vi "Message Update.vi"(8 "error in (no error)":errorcluster, 9 "Replace request":T1, 10 "Message type":string="Message") -> (0 "error out":errorcluster, 2 "Message Out":string)   [LabVIEW 2019]
uses:
  controls/Replace Request.ctl
  controls/Message_type.ctl
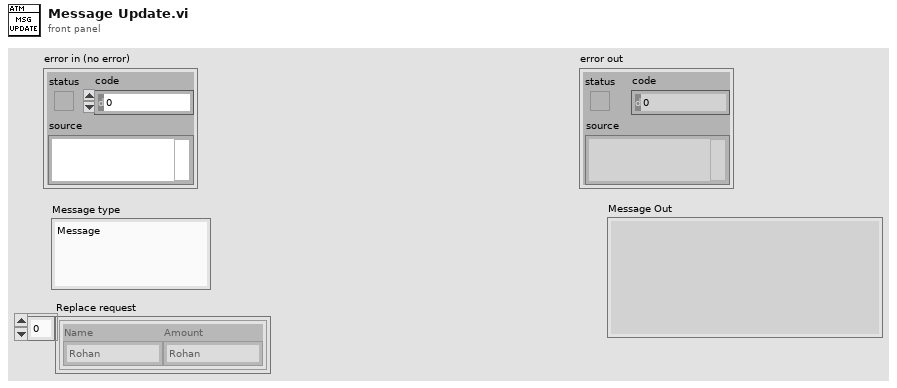
[diagram p1: front panel]
types:
  T1 = typedef "Replace Request.ctl" = cluster{"Name":string, "Amount":string}[]
  T2 = typedef "Message_type.ctl" = string[][]
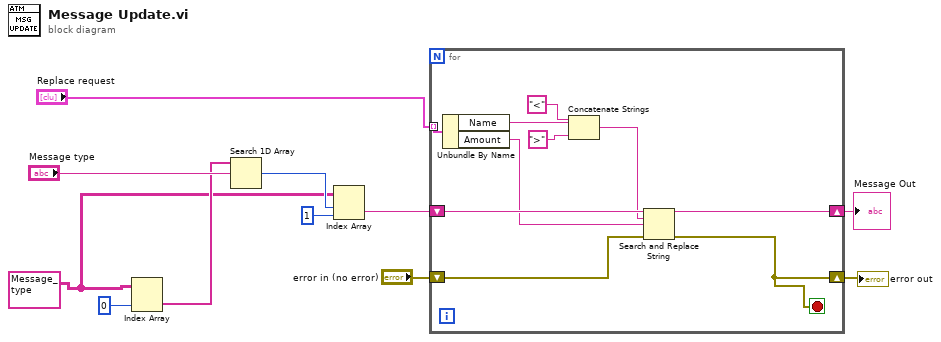
[diagram p0: block diagram]
diagram:
  w1 = T2 [["Welcome", "Welcome to Acme Bank.\nPlease insert your card\nand enter your account\nnumber in the User Input.\n\nPress Enter (E) when done."], ["Main Menu", "Welcome to Acme Bank\n<Name>\n\nPlease select transaction by using the buttons."], ["Account Verification Failed", "Account Information Incorrect.\nPlease Re-Enter Account Number.\nPress Enter (E) when done."], ["Session Terminate", "Your session has been terminated due to inactivity or menu selection.\nPlease take your card.\n\nGoodbye!"], ["Deposit", "Please enter amount to deposit and press Enter (E) when done."], ["Deposit Complete", "<Amount> Deposited"], ["Withdrawal", "Please enter amount to withdraw and press Enter (E) when done."], ["Withdrawal Complete", "<Amount> Withdrawn"], ["Withdrawal Failed", "Insufficient funds in account.\nPlease check your balance and try again."], ["Balance Inquiry", "Your Balance Is:\n<Amount>"]] ("Messages")
  n1 = Index Array(array=w1, index (col)=0 ("index (row)")) -> (element=w10:string[])  [unwired: 1 in]
  n2 = Search 1D Array(1D array=w10, element="Message type") -> (index of element=w6:i32)  [unwired: 1 in]
  n3 = Index Array(array=w1, index (row)=w6, index (col)=1 ("disabled index (col)")) -> (element=w4:string)
  n4 = for {
    shift-right: [w15] -> w8
    shift-left: "error in (no error)" -> [w16]
    shift-right: [w19] -> w3
    shift-left: w4 -> [w18]
    tunnel: "Replace request" -> [w14] mode=indexing
    stop <- w15 stop-if-true
    n5 = Unbundle By Name(w14) -> ("Name"=w13:string, "Amount"=w12:string)
    n6 = Concatenate Strings("<" ("string"), w13, ">" ("string")) -> (w17:string)
    n7 = Search and Replace String(input string=w18, search string=w17, replace string=w12, error in=w16) -> (result string=w19:string, error out=w15:errorcluster)  [unwired: 4 in, 2 out]
  }
  "error out" <- w8
  "Message Out" <- w3
